vi "MultiLogger.vi"() -> ()   [LabVIEW 2015]
doc: "This logs data to a comma separated text file which can be read into matlab by LVimport.m. Set the sample rate and the samples per buffer. A new measurement channel is created for every element in the channel array. Use context help for more info. <b> Measurements can only be made on a single device per instance of this VI </b>\n\nLove Jimbles"
uses:
  <vilib>/Utility/error.llb/DialogType.ctl
  <vilib>/DAQmx/read.llb/DAQmx Read (Analog 2D DBL NChan NSamp).vi
  <vilib>/DAQmx/create/channels.llb/DAQmx Create Channel (AI-Voltage-Basic).vi
  <vilib>/DAQmx/configure/timing.llb/DAQmx Timing (Sample Clock).vi
  <vilib>/DAQmx/miscellaneous.llb/DAQmx Fill In Error Info.vi
  <resource>/objmgr/daqmx.rc
panel:
  out "graph update time (s)":dbl
  in  "Channel Array":T1(array[cluster]) {"max value" format="%0.2f"; "min value" format="%0.2f"; "units" items=["Volts"=10348, "From Custom Scale"=10065]; "configuration" items=["RSE"=10083, "NRSE"=10078, "Differential"=10106, "Pseudodifferential"=12529]}
  in  "stop":bool
  out "Measurement":dbl[][](graph)
  in  "Samples to Read":i32=1000 caption="Samples per buffer" min=1 step=1000
  in  "Rate":dbl=1000.0 caption="Sample Rate (Hz)" min=0.0 step=1000.0 format="%0.2f"
  # "CONTEXT HELP (ctr+h) IS YOUR FRIEND"
  # "right click graph to autoscale Y axis"
  # "<<<<< THIS IS IMPORTANT"
  # "Add a channel by activating one of the controls.  Delete using right click > data operations > delete element"
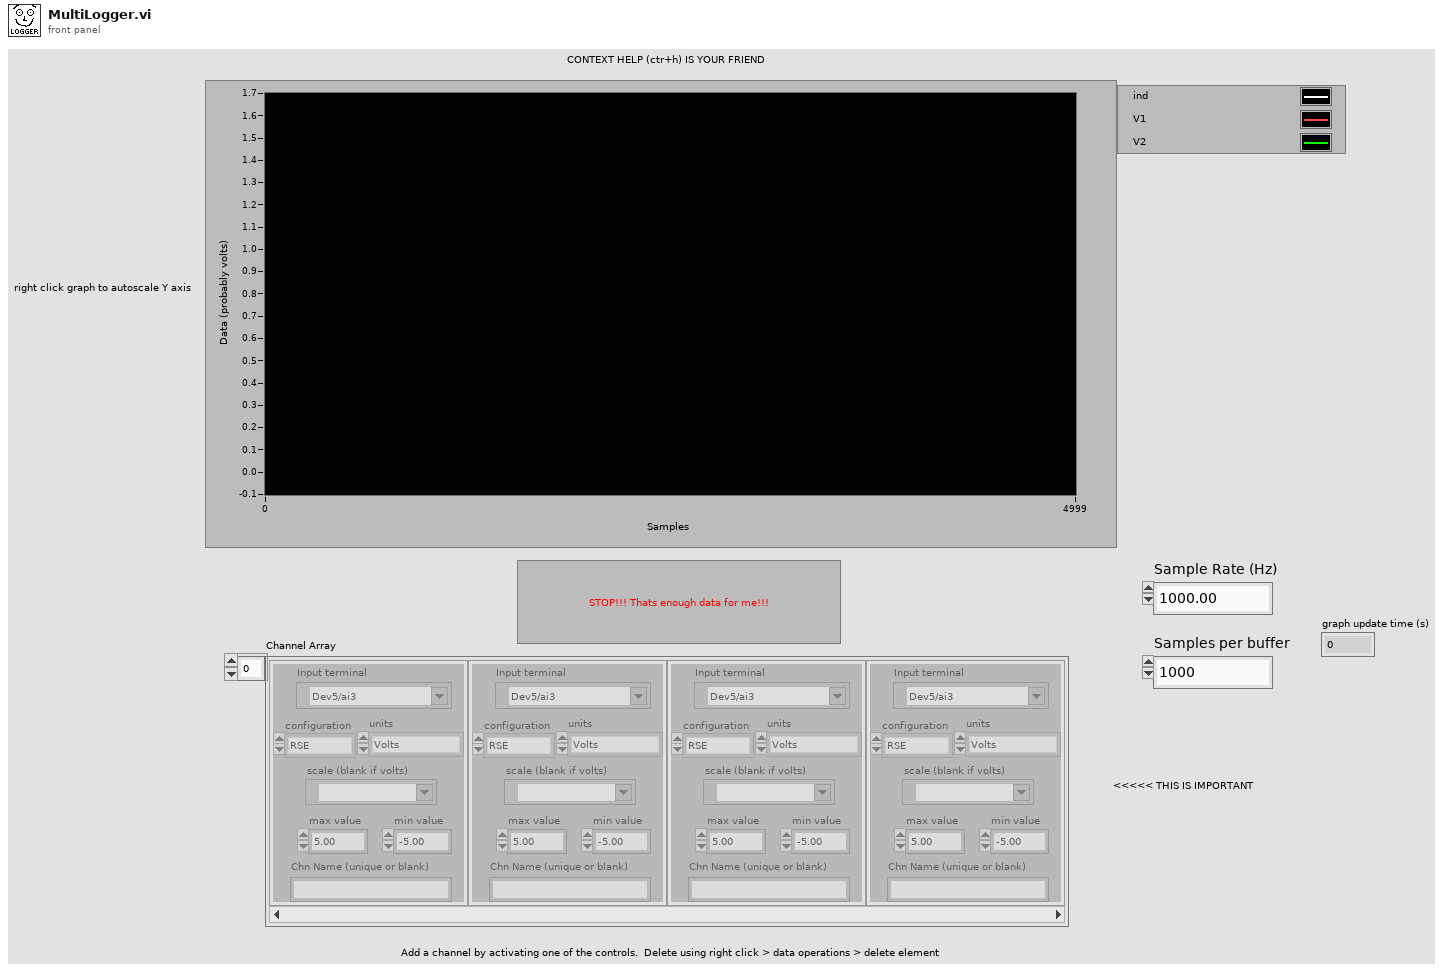
[diagram p1: front panel]
types:
  T1 = cluster{"Input terminal":tag, "configuration":i32, "units":i32, "min value":dbl, "max value":dbl, "Chn Name (unique or blank)":string, "scale (blank if volts)":tag}[]
  T2 = typedef "DialogType.ctl" = u16
  T3 = cluster{"Input terminal":tag, "configuration":i32, "units":i32, "min value":dbl, "max value":dbl, "Chn Name (unique or blank)":string, "scale (blank if volts)":tag}
  T4 = enum16{"Left Button", "Center Button", "Right Button", "Window Close"}
  T5 = enum16{"open", "replace", "create", "open or create", "replace or create", "replace or create with confirmation"}
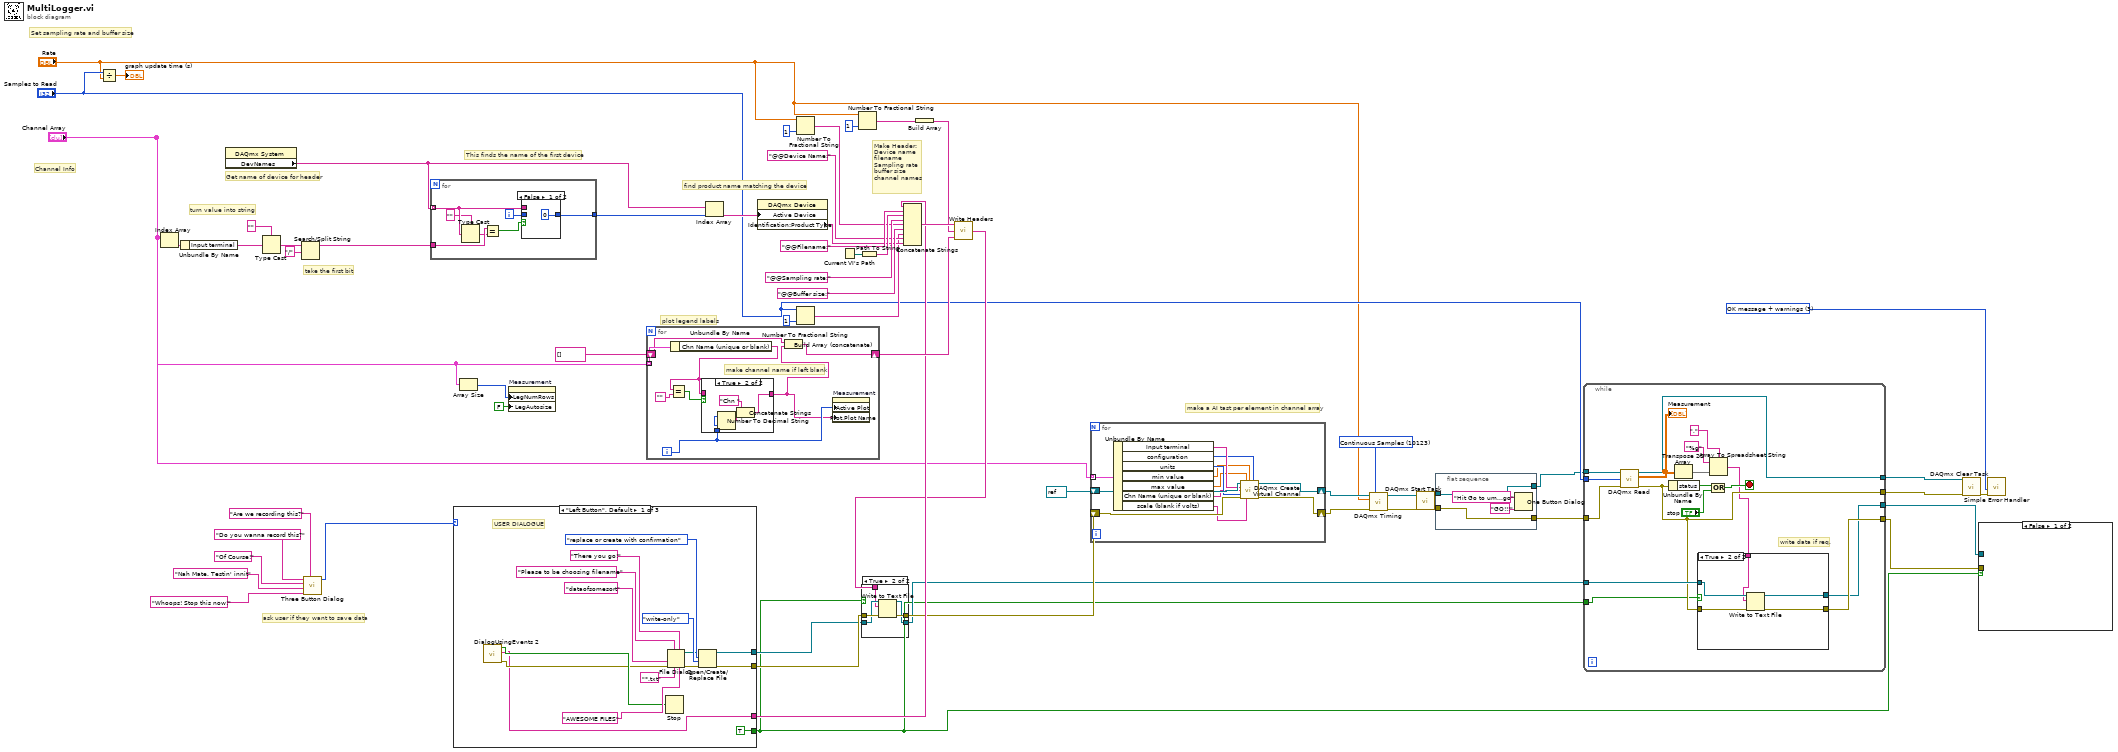
[diagram p0: block diagram]
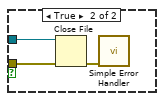
[diagram p3: hidden frame]
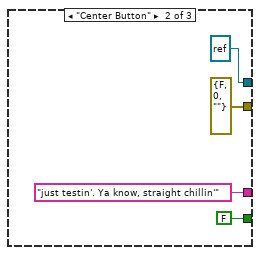
[diagram p4: hidden frame]
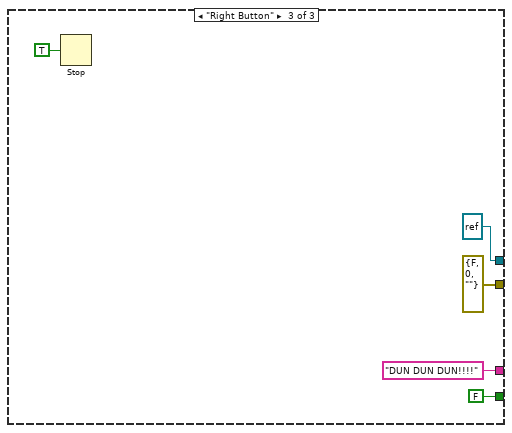
[diagram p5: hidden frame]
diagram:
  w59 = T2 3 items=["no dialog", "OK message", "continue or stop message", "OK message + warnings", "continue/stop + warnings"] ("type of dialog (OK msg:1)")
  w60 = 10123 items=["Finite Samples"=10178, "Continuous Samples"=10123] ("sample mode")
  # "make a AI tast per element in channel array"
  # "plot legend labels"
  # "ask user if they want to save data"
  # "find product name matching the device"
  # "take the first bit"
  # "turn value into string"
  # "Make Header:\nDevice name\nfilename\nSampling rate\nbuffer size\nchannel names"
  # "This finds the name of the first device"
  # "Channel Info"
  # "Set sampling rate and buffer size"
  # "Get name of device for header"
  n1 = Divide(x="Samples to Read", y="Rate") -> (x/y=→"graph update time (s)":dbl)
  n2 = Index Array(array="Channel Array") -> (element=w29:T3)  [unwired: 1 in]
  n3 = Unbundle By Name(w29) -> ("Input terminal"=w28:tag)
  n4 = property class="DAQmx System"() -> ("DevNames"=w35:tag[])  [unwired: 2 in, 2 out]
  n5 = Type Cast(type="", x=w28) -> (*(type *) &x=w41:string)
  n6 = Search/Split String(string=w41, search string/char (-)="/") -> (substring before match=w39:string)  [unwired: 1 in, 2 out]
  n7 = call <vilib>:"Three Button Dialog.vi"("Window Title (\"\")"="Are we recording this?" ("Window Title (\"\")"), "Right Button Text (\"Cancel\")"="Whoops! Stop this now!" ("Right Button Text (\"Cancel\")"), "Center Button Text (\"No\")"="Nah Mate. Testin' innit" ("Center Button Text (\"No\")"), "Left Button Text (\"Yes\")"="Of Course!" ("Left Button Text (\"Yes\")"), "message"="Do you wanna record this?") -> ("Which Button?"=w19:T4)  [unwired: 6 in]
  n8 = for {
    tunnel: w35 -> [w68] mode=indexing
    tunnel: w39 -> [w66]
    tunnel: [w63] -> w34
    i -> [w62]
    n9 = Type Cast(type="", x=w68) -> (*(type *) &x=w65:string)
    n10 = Equal?(x=w66, y=w65) -> (x = y?=w64:bool)
    n11 = case shown="False" w64 {
      tunnel: w68 -> [_ _]
      tunnel: [0 w70] -> w63
      tunnel: w62 -> [_ w70]
      frame False {
      }
      frame True {
      }
    }
  }
  n12 = case shown="\"Left Button\", Default" w19 {
    tunnel: [w71 "just testin'. Ya know, straight chillin'" ("Description") "DUN DUN DUN!!!!" ("Description")] -> w18
    tunnel: [w75 errorcluster {"status"=FALSE, "code"=0, "source"=""} ("error out") errorcluster {"status"=FALSE, "code"=0, "source"=""} ("error out")] -> w17
    tunnel: [w74 refnum<file> refnum ("refnum out") refnum<file> refnum ("refnum out")] -> w15
    tunnel: [TRUE FALSE FALSE] -> w13
    frame "Left Button", Default {
      # "USER DIALOGUE"
      n13 = call "DialogUsingEvents 2.vi"() -> ("error out"=w72:errorcluster, "Description 2"=w71:string, "Cancelled?"=w73:bool)  [unwired: 9 in]
      n14 = Stop(stop? (T)=w73) -> ()
      n15 = File Dialog(4:"AWESOME FILES" ("pattern label"), 5:"There you go!" ("button label"), 6:"*.txt" ("pattern (all files)"), 7:"Please to be choosing filename" ("prompt"), 8:w72, 9:"dataofsomesort" ("default name")) -> (0:w80:errorcluster, 3:w81:path)  [unwired: 3 out]
      n16 = Open/Create/Replace File(file path (use dialog)=w81, error in=w80, operation (0:open)=T5."replace or create with confirmation", access (0:read/write)=enum16{"read/write", "read-only", "write-only"}."write-only") -> (refnum out=w74:refnum<file>, error out=w75:errorcluster)  [unwired: 2 in, 1 out]
    }
    frame "Center Button" {
    }
    frame "Right Button" {
      n17 = Stop(stop? (T)=TRUE) -> ()
    }
  }
  n18 = Array Size(array="Channel Array") -> (size(s)=w10:i32)
  n19 = property on="Measurement" class="WFGraph (strict)"("LegNumRows"=w10, "LegAutosize"=FALSE ("Legend:Autosize")) -> ()  [unwired: 2 in, 2 out]
  n20 = for {
    tunnel: "Channel Array" -> [w102] mode=indexing
    shift-right: [w101] -> w25
    shift-left: string[] [] -> [w100]
    i -> [w96]
    # "make channel name if left blank"
    n21 = Unbundle By Name(w102) -> ("Chn Name (unique or blank)"=w99:string)
    n22 = Equal?(x=w99, y="") -> (x = y?=w97:bool)
    n23 = case shown="True" w97 {
      tunnel: [w103 w106] -> w95
      tunnel: w99 -> [w103 _]
      tunnel: w96 -> [_ w105]
      frame False {
      }
      frame True {
        n24 = Number To Decimal String(number=w105) -> (decimal integer string=w104:string)  [unwired: 1 in]
        n25 = Concatenate Strings("Chn ", w104) -> (w106:string)
      }
    }
    n26 = Build Array (concatenate)(w100, w95) -> (w101:string[])
    n27 = property on="Measurement" class="WFGraph (strict)"("Active Plot"=w96, "Plot.Plot Name"=w95) -> ()  [unwired: 2 in, 2 out]
  }
  n28 = Index Array(array=w35, index=w34) -> (element=w36:tag)
  n29 = property class="DAQmx Device"("Active Device"=w36) -> ("Identification:Product Type"=w37:string)  [unwired: 2 in, 2 out]
  n30 = Number To Fractional String(number="Rate", precision (6)=i16 1) -> (F-format string=w47:string)  [unwired: 2 in]
  n31 = Number To Fractional String(number="Samples to Read", precision (6)=i16 1) -> (F-format string=w33:string)  [unwired: 2 in]
  n32 = Current VI's Path() -> (path=w53:path)
  n33 = Number To Fractional String(number="Rate", precision (6)=i16 1) -> (F-format string=w45:string)  [unwired: 2 in]
  n34 = Path To String(path=w53) -> (string=w51:string)
  n35 = Concatenate Strings(w18, "@@Filename:" ("string"), w51, "@@Sampling rate:" ("string"), w47, "@@Buffer size:" ("string"), w33, "@@Device Name:" ("string"), w37) -> (w54:string)
  n36 = Build Array(w45) -> (w49:string[])
  n37 = call "Write Headers.vi"("Channel Names"=w25, "Sampling Rates"=w49, "Description"=w54) -> ("Full Header String"=w12:string)
  n38 = case shown="True" w13 {
    tunnel: w17 -> [w108 w114]
    tunnel: [w108 w113] -> w16
    tunnel: w15 -> [w109 w112]
    tunnel: [w109 w111] -> w14
    tunnel: w12 -> [_ w110]
    frame False {
    }
    frame True {
      n39 = Write to Text File(file (use dialog)=w112, text=w110, error in=w114) -> (refnum out=w111:refnum<file>, error out=w113:errorcluster)  [unwired: 1 in, 1 out]
    }
  }
  n40 = for {
    shift-right: [w125] -> w31
    shift-left: w16 -> [w126]
    shift-right: [w124] -> w30
    shift-left: refnum<k21> refnum ("task out") -> [w123]
    tunnel: "Channel Array" -> [w122] mode=indexing
    n41 = Unbundle By Name(w122) -> ("Input terminal"=w121:tag, "configuration"=w120:i32, "units"=w119:i32, "min value"=w118:dbl, "max value"=w117:dbl, "Chn Name (unique or blank)"=w116:string, "scale (blank if volts)"=w115:tag)
    n42 = call-poly <vilib>:"DAQmx Create Virtual Channel.vi"("task in"=w123, "maximum value"=w117, "minimum value"=w118, "input terminal configuration"=w120, "physical channels"=w121, "name to assign"=w116, "units"=w119, "error in"=w126, "custom scale name"=w115) -> ("task out"=w124:refnum<k21>, "error out"=w125:errorcluster)  [unwired: 5 in]
  }
  n43 = call-poly <vilib>:"DAQmx Timing.vi"("task/channels in"=w30, "sample mode"=w60, "rate"="Rate", "error in"=w31) -> ("task out"=w5:refnum<k21>, "error out"=w50:errorcluster)  [unwired: 10 in]
  n44 = call <vilib>:"DAQmx Start Task.vi"("task/channels in"=w5, "error in"=w50) -> ("task out"=w3:refnum<k21>, "error out"=w4:errorcluster)  [unwired: 12 in]
  n45 = flat-sequence {
    tunnel: w4 -> [w129]
    tunnel: w3 -> [w130]
    tunnel: [w130] -> w2
    tunnel: [w129] -> w1
    frame #0 {
      n46 = One Button Dialog(message="Hit Go to um...go", button name ("OK")="GO!!!") -> ()  [unwired: 1 out]
    }
  }
  n47 = while {
    tunnel: [w136] -> w57
    tunnel: w2 -> [w147]
    tunnel: [w146] -> w58
    tunnel: w14 -> [w137]
    tunnel: [w134] -> w56
    tunnel: [w135] -> w55
    tunnel: "Samples to Read" -> [w142]
    tunnel: w13 -> [w132]
    tunnel: w1 -> [w131]
    stop <- w143 stop-if-true
    # "write data if req."
    n48 = call-poly <vilib>:"DAQmx Read.vi"("task/channels in"=w147, "number of samples per channel"=w142, "error in"=w131) -> ("task out"=w146:refnum<k21>, "data"=w139:dbl[][], "error out"=w136:errorcluster)  [unwired: 10 in]
    "Measurement" <- w139
    n49 = Unbundle By Name(w136) -> ("status"=w145:bool)
    n50 = Transpose 2D Array(2D array=w139) -> (transposed array=w138:dbl[][])
    n51 = Array To Spreadsheet String(delimiter (Tab)=",", array=w138, 3:"%g" ("format string")) -> (spreadsheet string=w133:string)
    n52 = case shown="True" w132 {
      tunnel: w137 -> [w149 w154]
      tunnel: w136 -> [w148 w153]
      tunnel: [w148 w152] -> w135
      tunnel: [w149 w151] -> w134
      tunnel: w133 -> [_ w150]
      frame False {
      }
      frame True {
        n53 = Write to Text File(file (use dialog)=w154, text=w150, error in=w153) -> (refnum out=w151:refnum<file>, error out=w152:errorcluster)  [unwired: 1 in, 1 out]
      }
    }
    n54 = Compound Arithmetic op=OR(w145, "stop") -> (w143:bool)
  }
  n55 = call <vilib>:"DAQmx Clear Task.vi"("task in"=w58, "error in"=w57) -> ("error out"=w61:errorcluster)  [unwired: 13 in]
  n56 = case shown="False" w13 {
    tunnel: w56 -> [_ w156]
    tunnel: w55 -> [_ w155]
    frame False {
    }
    frame True {
      n57 = Close File(refnum=w156, error in=w155) -> (error out=w157:errorcluster)  [unwired: 1 out]
      n58 = call <vilib>:"Simple Error Handler.vi"("error in (no error)"=w157) -> ()  [unwired: 4 in, 5 out]
    }
  }
  n59 = call <vilib>:"Simple Error Handler.vi"("type of dialog (OK msg:1)"=w59, "error in (no error)"=w61) -> ()  [unwired: 3 in, 5 out]
